vi "Read ackCMDEvent.vi"(8 "error in (no error)":errorcluster, 11 "PubSubDataEvent in":refnum<class "PubSubDataEvent.lvclass">) -> (0 "error out":errorcluster, 2 "ackCMDEvent":cluster{"ackCMD":refnum<user-event>}, 3 "PubSubDataEvent out":refnum<class "PubSubDataEvent.lvclass">)   [LabVIEW 2016, in "PubSubDataEvent.lvclass"]
uses:
  PubSubDataEvent.lvclass
  Typedefs/CommandValue.ctl
  PubSubDataEvent.lvclass/PubSubDataEvent.ctl
  Typedefs/SEDSpectrometerTypedefs.lvlib
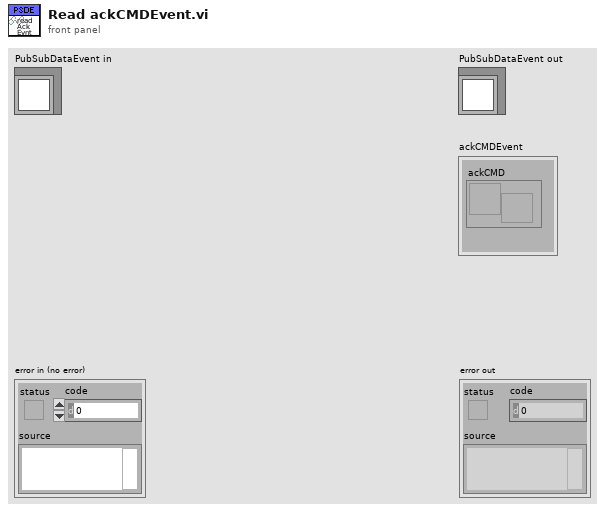
[diagram p1: front panel]
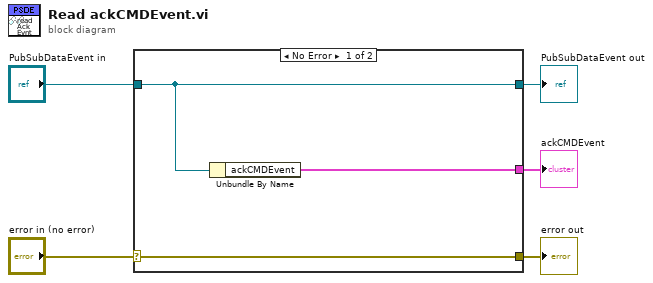
[diagram p0: block diagram]
diagram:
  n1 = case shown="No Error" "error in (no error)" {
    selector: "error in (no error)" -> [w8 w9]
    tunnel: [w8 w9] -> w4
    tunnel: [w7 w10] -> w2
    tunnel: "PubSubDataEvent in" -> [w7 w10]
    tunnel: [w6 _] -> w1
    frame No Error {
      n2 = Unbundle By Name(w7) -> ("ackCMDEvent"=w6:cluster{"ackCMD":refnum<user-event>})
    }
    frame Error {
    }
  }
  "error out" <- w4
  "PubSubDataEvent out" <- w2
  "ackCMDEvent" <- w1
